vi "add_pose.vi"(4 "Pose":T1, 5 "msg in":string) -> (2 "msg out":string)   [LabVIEW 2013]
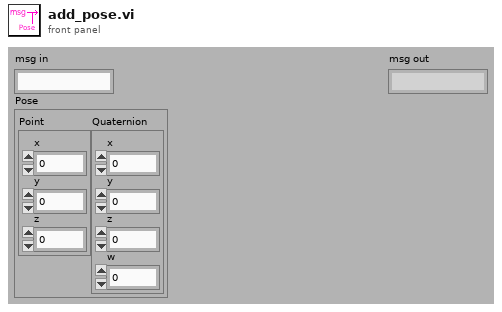
[diagram p1: front panel]
types:
  T1 = cluster{"Point":cluster{"x":dbl, "y":dbl, "z":dbl}, "Quaternion":cluster{"x":dbl, "y":dbl, "z":dbl, "w":dbl}}
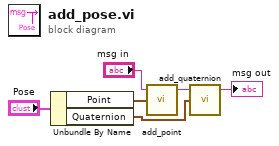
[diagram p0: block diagram]
diagram:
  n1 = Unbundle By Name("Pose") -> ("Point"=w4:cluster{"x":dbl, "y":dbl, "z":dbl}, "Quaternion"=w3:cluster{"x":dbl, "y":dbl, "z":dbl, "w":dbl})
  n2 = call "add_point.vi"("Point"=w4, "msg in"="msg in") -> ("msg out"=w6:string)  [unwired: 3 in]
  n3 = call "add_quaternion.vi"("Quaternion"=w3, "msg in"=w6) -> ("msg out"=→"msg out":string)  [unwired: 3 in]
